vi "Decode_SignedThousandths.vi"(1 "Little Endian":u8[](array[numeric])) -> (0 "Signed Thousandths (0.000)":dbl[](array[numeric]))   [LabVIEW 2015, in "navX Library v3.lvlib" / "navX Registry Cache.lvclass"]
uses:
  navX Registry Cache.lvclass
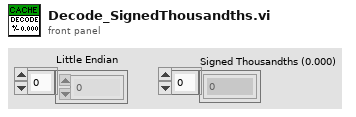
[diagram p1: front panel]
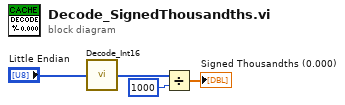
[diagram p0: block diagram]
diagram:
  n1 = call "Decode_Int16.vi"("Little Endian"="Little Endian") -> ("Int16"=w2:i16[])
  n2 = Divide(x=w2, y=1000) -> (x/y=→"Signed Thousandths (0.000)":dbl[])
